vi "Get Sensor Move In Previous.vi"(8 "error in (no error)":errorcluster, 11 "Abstract Sensor Move In Previous Msg in":refnum<class "Abstract Sensor Move In Previous Msg.lvclass">) -> (0 "error out":errorcluster, 2 "Sensor Move In Previous":bool, 3 "Abstract Sensor Move In Previous Msg out":refnum<class "Abstract Sensor Move In Previous Msg.lvclass">)   [LabVIEW 2013, in "Sensor Model.lvlib" / "Abstract Sensor Move In Previous Msg.lvclass"]
uses:
  Abstract Sensor Move In Previous Msg.lvclass
  Abstract Sensor Move In Previous Msg.lvclass/Abstract Sensor Move In Previous Msg.ctl
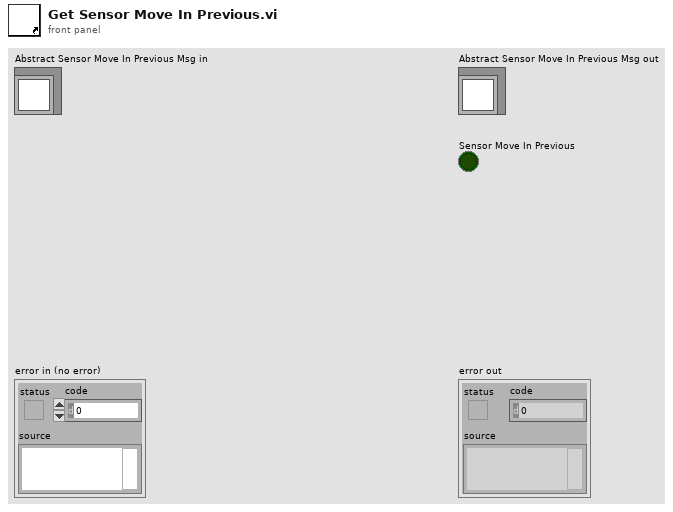
[diagram p1: front panel]
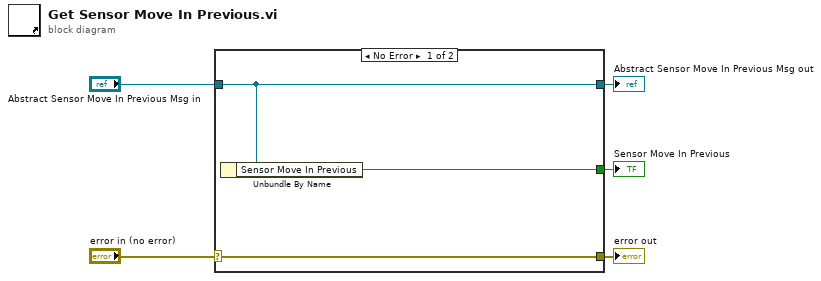
[diagram p0: block diagram]
diagram:
  n1 = case shown="No Error" "error in (no error)" {
    selector: "error in (no error)" -> [w8 w9]
    tunnel: [w8 w9] -> w4
    tunnel: [w7 w10] -> w2
    tunnel: "Abstract Sensor Move In Previous Msg in" -> [w7 w10]
    tunnel: [w6 _] -> w1
    frame No Error {
      n2 = Unbundle By Name(w7) -> ("Sensor Move In Previous"=w6:bool)
    }
    frame Error {
    }
  }
  "error out" <- w4
  "Abstract Sensor Move In Previous Msg out" <- w2
  "Sensor Move In Previous" <- w1
